vi "Device Select.vi"(8 "error in (no error)":errorcluster, 10 "SQL query":string="SELECT distinct DeviceName \nFROM\nltt.daq_configuration\n Where ChannelType='PWM_Output' and Enabled=1;", 11 "PWM Output in":refnum<class "PWM Output.lvclass">) -> (0 "error out":errorcluster, 3 "PWM Output out":refnum<class "PWM Output.lvclass">)   [LabVIEW 2023, in "HardwareAbstractionLayer_LVOOP.lvlib" / "PWM Output.lvclass"]
uses:
  PWM Output.lvclass
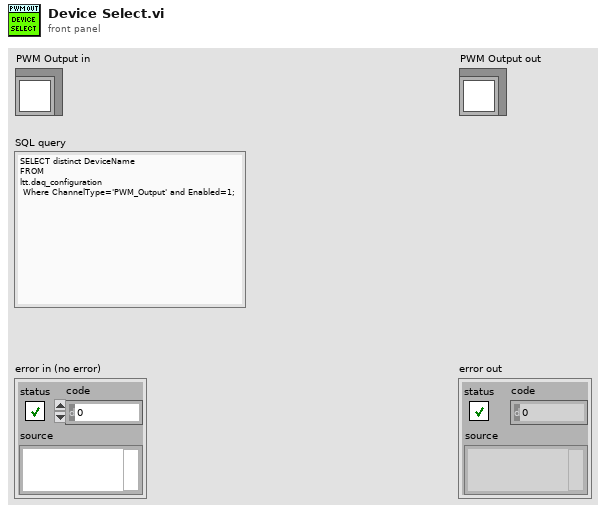
[diagram p1: front panel]
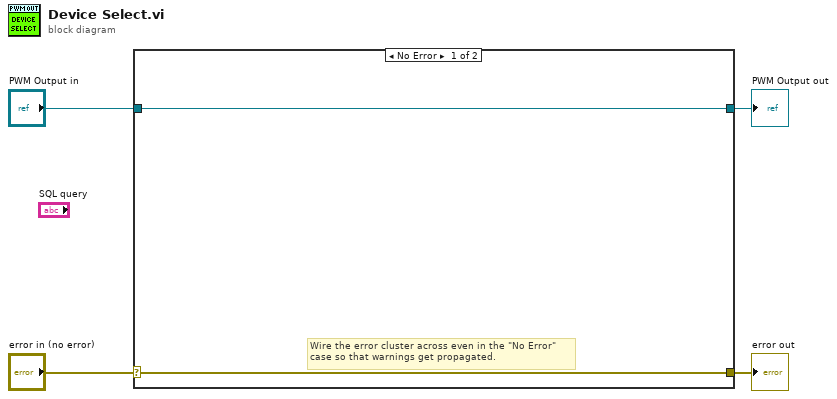
[diagram p0: block diagram]
diagram:
  n1 = case shown="No Error" "error in (no error)" {
    selector: "error in (no error)" -> [w5 w8]
    tunnel: [w5 w8] -> w3
    tunnel: [w6 w7] -> w1
    tunnel: "PWM Output in" -> [w6 w7]
    frame No Error {
      # "Wire the error cluster across even in the \"No Error\"\ncase so that warnings get propagated."
    }
    frame Error {
    }
  }
  "error out" <- w3
  "PWM Output out" <- w1
